vi "Init_UI_Cluster.vi"(8 "error in (no error)":errorcluster, 11 "Cluster_IN":T1) -> (0 "error out":errorcluster, 3 "Cluster_OUT":T1)   [LabVIEW 2020]
uses:
  Controls/UI_Cluster.ctl
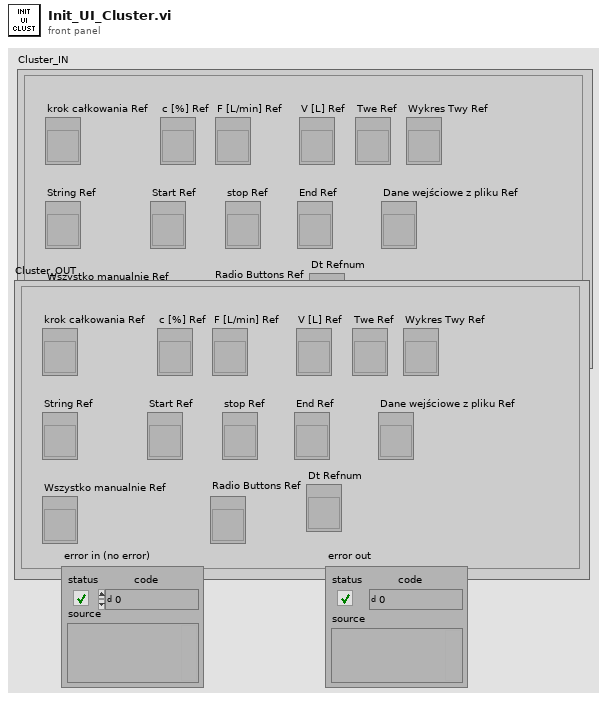
[diagram p1: front panel]
types:
  T1 = typedef "UI_Cluster.ctl" = cluster{"krok całkowania Ref":refnum<vi>, "c [%] Ref":refnum<vi>, "F [L/min] Ref":refnum<vi>, "V [L] Ref":refnum<vi>, "Twe Ref":refnum<vi>, "Wykres Twy Ref":refnum<vi>, "String Ref":refnum<vi>, "Start Ref":refnum<vi>, "stop Ref":refnum<vi>, "End Ref":refnum<vi>, "Dane wejściowe z pliku Ref":refnum<vi>, "Wszystko manualnie Ref":refnum<vi>, "Dt Refnum":refnum<vi>, "Radio Buttons Ref":refnum<vi>}
  T2 = enum8{"Enabled", "Disabled", "Disabled and Grayed Out"}
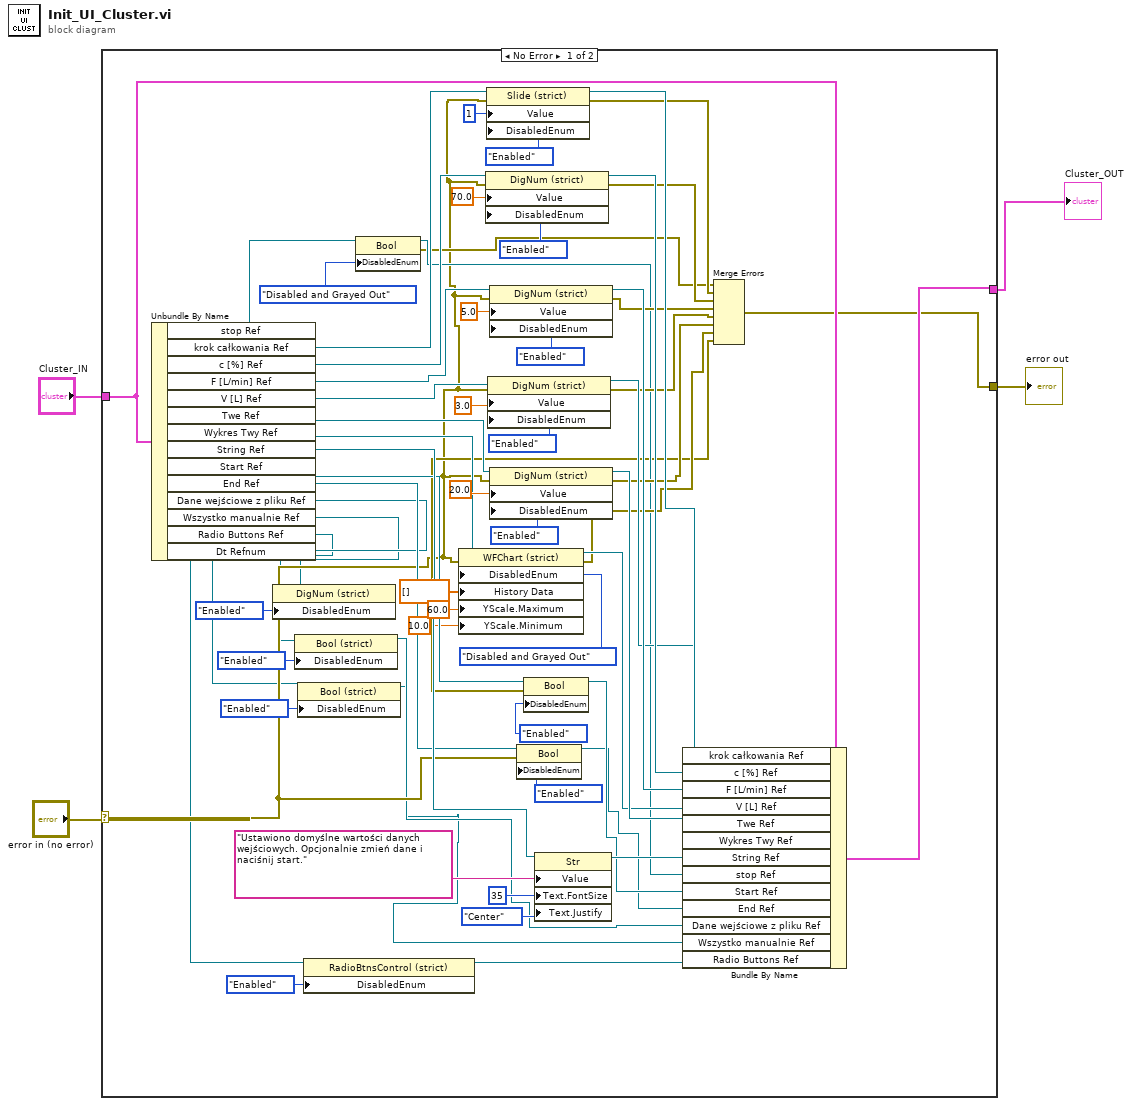
[diagram p0: block diagram]
diagram:
  n1 = case shown="No Error" "error in (no error)" {
    selector: "error in (no error)" -> [w21 w68]
    tunnel: "Cluster_IN" -> [w59 w69]
    tunnel: [w48 w69] -> w2
    tunnel: [w41 w68] -> w1
    frame No Error {
      n2 = Unbundle By Name(w59) -> ("stop Ref"=w30:refnum<vi>, "krok całkowania Ref"=w67:refnum<vi>, "c [%] Ref"=w65:refnum<vi>, "F [L/min] Ref"=w56:refnum<vi>, "V [L] Ref"=w63:refnum<vi>, "Twe Ref"=w61:refnum<vi>, "Wykres Twy Ref"=w51:refnum<vi>, "String Ref"=w40:refnum<vi>, "Start Ref"=w26:refnum<vi>, "End Ref"=w22:refnum<vi>, "Dane wejściowe z pliku Ref"=w17:refnum<vi>, "Wszystko manualnie Ref"=w15:refnum<vi>, "Radio Buttons Ref"=w11:refnum<vi>, "Dt Refnum"=w6:refnum<vi>)
      n3 = property class="DigNum (strict)"(reference=w6, "DisabledEnum"=T2."Enabled" ("Disabled")) -> ()  [unwired: 1 in, 2 out]
      n4 = property class="Bool (strict)"(reference=w17, "DisabledEnum"=T2."Enabled" ("Disabled")) -> (reference out=w13:refnum<vi>)  [unwired: 1 in, 1 out]
      n5 = property class="Bool (strict)"(reference=w15, "DisabledEnum"=T2."Enabled" ("Disabled")) -> (reference out=w12:refnum<vi>)  [unwired: 1 in, 1 out]
      n6 = property class="RadioBtnsControl (strict)"(reference=w11, "DisabledEnum"=T2."Enabled" ("Disabled")) -> (reference out=w9:refnum<vi>)  [unwired: 1 in, 1 out]
      n7 = property class="Bool"(reference=w30, "DisabledEnum"=T2."Disabled and Grayed Out" ("Disabled")) -> (reference out=w28:refnum<vi>, error out=w27:errorcluster)  [unwired: 1 in]
      n8 = property class="WFChart (strict)"(reference=w51, error in=w21, "DisabledEnum"=T2."Disabled and Grayed Out" ("Disabled"), "History Data"=dbl[] [], "YScale.Maximum"=60.0 ("Y Scale.Range:Maximum"), "YScale.Minimum"=10.0 ("Y Scale.Range:Minimum")) -> (reference out=w49:refnum<vi>, error out=w42:errorcluster)
      n9 = property class="DigNum (strict)"(reference=w65, error in=w21, "Value"=70.0, "DisabledEnum"=T2."Enabled" ("Disabled")) -> (reference out=w57:refnum<vi>, error out=w46:errorcluster)
      n10 = property class="Slide (strict)"(reference=w67, error in=w21, "Value"=u32 1, "DisabledEnum"=T2."Enabled" ("Disabled")) -> (reference out=w58:refnum<vi>, error out=w47:errorcluster)
      n11 = property class="DigNum (strict)"(reference=w63, error in=w21, "Value"=3.0, "DisabledEnum"=T2."Enabled" ("Disabled")) -> (reference out=w53:refnum<vi>, error out=w44:errorcluster)
      n12 = property class="DigNum (strict)"(reference=w56, error in=w21, "Value"=5.0, "DisabledEnum"=T2."Enabled" ("Disabled")) -> (reference out=w54:refnum<vi>, error out=w45:errorcluster)
      n13 = property class="DigNum (strict)"(reference=w61, error in=w21, "Value"=20.0, "DisabledEnum"=T2."Enabled" ("Disabled")) -> (reference out=w52:refnum<vi>, error out=w43:errorcluster)
      n14 = property class="Bool"(reference=w22, error in=w21, "DisabledEnum"=T2."Enabled" ("Disabled")) -> (reference out=w19:refnum<vi>)  [unwired: 1 out]
      n15 = property class="Bool"(reference=w26, "DisabledEnum"=T2."Enabled" ("Disabled")) -> (reference out=w24:refnum<vi>, error out=w23:errorcluster)  [unwired: 1 in]
      n16 = property class="Str"(reference=w40, "Value"="Ustawiono domyślne wartości danych wejściowych. Opcjonalnie zmień dane i naciśnij start.", "Text.FontSize"=u32 35 ("Text.Font:Size"), "Text.Justify"=enum16{"Left", "Center", "Right"}."Center" ("Text.Justification")) -> (reference out=w38:refnum<vi>)  [unwired: 1 in, 1 out]
      n17 = Bundle By Name(cluster=w59, "krok całkowania Ref"=w58, "c [%] Ref"=w57, "F [L/min] Ref"=w54, "V [L] Ref"=w53, "Twe Ref"=w52, "Wykres Twy Ref"=w49, "String Ref"=w38, "stop Ref"=w28, "Start Ref"=w24, "End Ref"=w19, "Dane wejściowe z pliku Ref"=w13, "Wszystko manualnie Ref"=w12, "Radio Buttons Ref"=w9) -> (w48:T1)
      n18 = Merge Errors(w27, w47, w46, w45, w44, w43, w42, w23) -> (w41:errorcluster)
    }
    frame Error {
    }
  }
  "Cluster_OUT" <- w2
  "error out" <- w1
